vi "get type.vi"(1 "RIO Device":T1) -> (0 "Product Name":string)   [LabVIEW 2021]
uses:
  <vilib>/userdefined/Silver/nirio_resource_slv.ctl
  <vilib>/nisyscfg/Filter Mode.ctl
  <resource>/objmgr/nicontrollersysapi.rc
  <vilib>/nisyscfg/nisyscfg.lvlib
  <resource>/objmgr/niflexrioatomicsae.rc
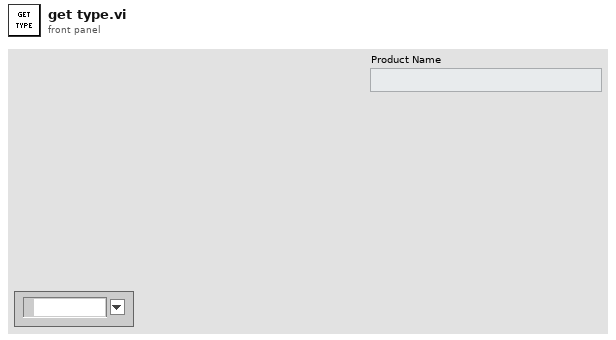
[diagram p1: front panel]
types:
  T1 = typedef "nirio_resource_slv.ctl" = tag
  T2 = typedef "nisyscfg.lvlib/Filter Mode.ctl" = i32
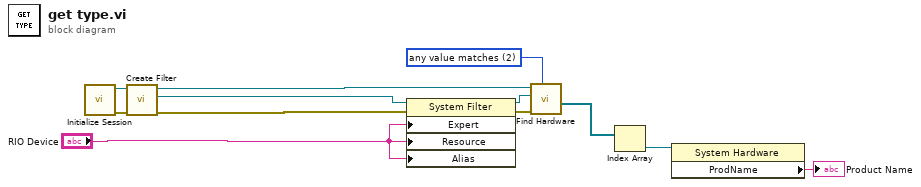
[diagram p0: block diagram]
diagram:
  w5 = T2 2 items=["all values match"=1, "any value matches"=2, "values do not match"=3, "all properties exist"=4] ("Filter Mode (all values match)")
  n1 = call <vilib>:"Initialize Session.vi"() -> ("error out"=w10:errorcluster, "Session out"=w11:refnum<k21>)  [unwired: 10 in]
  n2 = call <vilib>:"Create Filter.vi"("error in (no error)"=w10, "Session in"=w11) -> ("error out"=w8:errorcluster, "Filter out"=w9:refnum<k20>, "Session out"=w12:refnum<k21>)  [unwired: 7 in]
  n3 = property class="System Filter"(reference=w9, error in=w8, "Expert"="RIO Device", "Resource"="RIO Device", "Alias"="RIO Device") -> (reference out=w7:refnum<k20>, error out=w6:errorcluster)
  n4 = call <vilib>:"Find Hardware.vi"("Filter Mode (all values match)"=w5, "error in (no error)"=w6, "Filter in"=w7, "Session in"=w12) -> ("Resources out"=w4:refnum<k20>[])  [unwired: 7 out]
  n5 = Index Array(array=w4) -> (element=w3:refnum<k20>)  [unwired: 1 in]
  n6 = property class="System Hardware"(reference=w3) -> ("ProdName"=→"Product Name":string)  [unwired: 1 in, 2 out]
